vi "DigitalSignals.vi"(4 "PXITrigLaserClk":u8, 5 "LaserClkDelay":u8, 6 "Ref Clk Decimation":u8=25, 7 "PXITrigExtStartTrig":u8, 10 "AcqSoftStartTrig":bool, 11 "data in":T1={"channel 0"=[0, 0], "channel 1"=[0, 0], "channel 2"=[0, 0], "channel 3"=[0, 0], "channel 4"=[0, 0], "channel 5"=[0, 0], "channel 6"=[0, 0], "channel 7"=[0, 0]}) -> (2 "Digital Signals":cluster{"StartTrig":bool, "LaserClk":bool}, 3 "data out":T1)   [LabVIEW 2015]
uses:
  <vilib>/rvi/eio/common/nirviEmuTemplateMethod_errors.vi
  <vilib>/eio/EIONode/EIONode.xnode
  <vilib>/eio/EIOMethodNode/EIOMethodNode.xnode
  <vilib>/rvi/FXPMathLib/basic elements/FxpDiscreteDelay/XNode/nifxpmath_DiscreteDelay.xnode
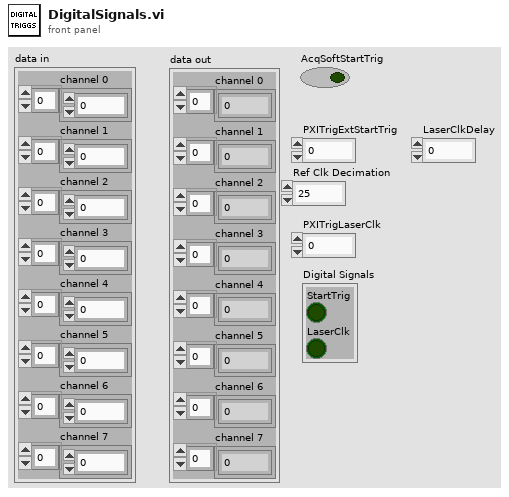
[diagram p1: front panel]
types:
  T1 = cluster{"channel 0":i16[], "channel 1":i16[], "channel 2":i16[], "channel 3":i16[], "channel 4":i16[], "channel 5":i16[], "channel 6":i16[], "channel 7":i16[]}
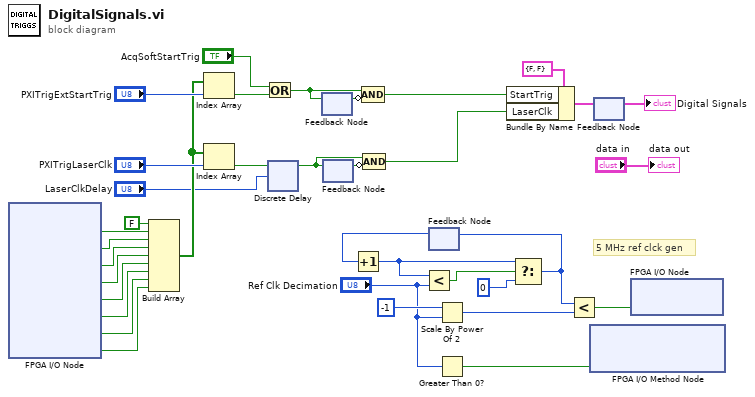
[diagram p0: block diagram]
diagram:
  # "5 MHz ref clck gen"
  n1 = xnode "FPGA I/O Node"() -> ("PXI_Trig0"=w33:bool, "PXI_Trig1"=w32:bool, "PXI_Trig2"=w31:bool, "PXI_Trig3"=w30:bool, "PXI_Trig4"=w29:bool, "PXI_Trig5"=w28:bool, "PXI_Trig6"=w27:bool, "PXI_Trig7"=w26:bool)  [unwired: 8 in, 8 out]
  n2 = Build Array(FALSE ("element"), w33, w32, w31, w30, w29, w28, w27, w26) -> (w19:bool[])
  n3 = Index Array(array=w19, index="PXITrigExtStartTrig") -> (element=w20:bool)
  n4 = Index Array(array=w19, index="PXITrigLaserClk") -> (element=w14:bool)
  n5 = Or(x="AcqSoftStartTrig", y=w20) -> (x .or. y?=w21:bool)
  n6 = xnode ("Discrete Delay")("D"=w14, "n-1[0..149]"="LaserClkDelay") -> ("Q"=w13:bool)
  n7 = feedback #1() -> (w34:bool)  [unwired: 1 in]
  n8 = feedback-in #1(w21) -> ()
  n9 = feedback #2() -> (w36:bool)  [unwired: 1 in]
  n10 = feedback-in #2(w13) -> ()
  n11 = Compound Arithmetic op=AND(w21, invert w34) -> (w16:bool)
  n12 = Compound Arithmetic op=AND(w13, invert w36) -> (w18:bool)
  n13 = feedback #3() -> (w6:u8)  [unwired: 1 in]
  n14 = Increment(x=w6) -> (x+1=w9:u8)
  n15 = Less?(x=w9, y="Ref Clk Decimation") -> (x < y?=w8:bool)
  n16 = Scale By Power Of 2(n=i16 -1, x="Ref Clk Decimation") -> (x*2^n=w4:u8)
  n17 = Greater Than 0?(x="Ref Clk Decimation") -> (x > 0?=w1:bool)
  n18 = Bundle By Name(cluster=cluster{"StartTrig":bool, "LaserClk":bool} {"StartTrig"=FALSE, "LaserClk"=FALSE}, "StartTrig"=w16, "LaserClk"=w18) -> (w15:cluster{"StartTrig":bool, "LaserClk":bool})
  n19 = Select(t=w9, s=w8, f=u8 0) -> (s? t:f=w7:u8)
  n20 = feedback-in #3(w7) -> ()
  n21 = Less?(x=w7, y=w4) -> (x < y?=w5:bool)
  n22 = xnode "FPGA I/O Method Node"("Enable"=w1) -> ()  [unwired: 1 in, 1 out]
  n23 = feedback-in #4(w15) -> ()
  n24 = feedback #4() -> (→"Digital Signals":cluster{"StartTrig":bool, "LaserClk":bool})  [unwired: 1 in]
  n25 = xnode "FPGA I/O Node"("PXI_Trig7"=w5) -> ()  [unwired: 1 in, 1 out]
  "data out" <- "data in"
